vi "Start Async.vi"(8 "error in (no error)":errorcluster, 11 "gRPC service in":refnum<class "MeasurementServiceBaseV2.lvclass">) -> (0 "error out":errorcluster, 3 "gRPC service out":refnum<class "MeasurementServiceBaseV2.lvclass">)   [LabVIEW 2021, in "ni.measurementlink.measurement.v2.api.lvlib" / "MeasurementServiceBaseV2.lvclass"]
uses:
  MeasurementServiceBaseV2.lvclass
  MeasurementServiceBaseV2.lvclass/MeasurementServiceBaseV2.ctl
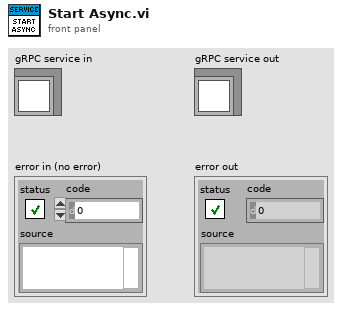
[diagram p1: front panel]
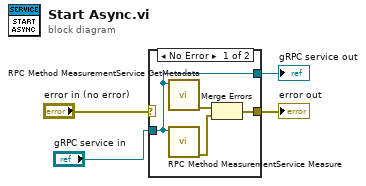
[diagram p0: block diagram]
diagram:
  n1 = case shown="No Error" "error in (no error)" {
    selector: "error in (no error)" -> [_ w10]
    tunnel: [w8 w10] -> w3
    tunnel: [w7 w9] -> w1
    tunnel: "gRPC service in" -> [w7 w9]
    frame No Error {
      n2 = call "RPC Method MeasurementService GetMetadata.vi"("gRPC service in"=w7) -> ("error out"=w6:errorcluster)  [unwired: 9 in, 1 out]
      n3 = call "RPC Method MeasurementService Measure.vi"("gRPC service in"=w7) -> ("error out"=w5:errorcluster)  [unwired: 9 in, 1 out]
      n4 = Merge Errors(w6, w5) -> (w8:errorcluster)
    }
    frame Error {
    }
  }
  "error out" <- w3
  "gRPC service out" <- w1
